vi "Test App Error Handler is Configured for Immediate Parent of Nested Process.vi"(8 "error in (no error)":errorcluster, 11 "Rig Test In":refnum<class "Application Test.lvclass">) -> (0 "error out":errorcluster, 3 "Rig Test Out":refnum<class "Application Test.lvclass">)   [LabVIEW 2020, in "Application Test.lvclass"]
uses:
  Application Test.lvclass
  Framework/Process/Process.lvclass
  Mock Error Handler/Mock Error Handler.lvclass
  Mock Process/Mock Process.lvclass
  Framework/Application/Application.lvclass
  <vilib>/Asteme/LUnit/Test Case.lvclass
  C:/Users/anton/Documents/GitHub/Triarc-Framework/source/Framework/Process/Process.lvclass
  C:/Users/anton/Documents/GitHub/Triarc-Framework/source/Framework/Base/Base.lvclass
  C:/Users/anton/Documents/GitHub/Triarc-Framework/source/Framework/Error Handler Interface/Error Handler Interface.lvclass
  C:/Users/anton/Documents/GitHub/Triarc-Framework/source/Framework/Logging/Logging.lvclass
  C:/Users/anton/Documents/GitHub/Triarc-Framework/source/Framework/Application/Application.lvclass
  C:/Users/anton/Documents/GitHub/Triarc-Framework/source/Framework Test/Process Test/Process Test.lvclass
  C:/Users/anton/Documents/GitHub/Triarc-Framework/source/Framework Test/Base Class Test/Base Test.lvclass
  C:/Program Files (x86)/National Instruments/LabVIEW 2020/vi.lib/Asteme/LUnit/Test Case.lvclass
  C:/Users/anton/Documents/GitHub/Triarc-Framework/source/Framework Test/Application Test/Application Test.lvclass
  C:/Users/anton/Documents/GitHub/Triarc-Framework/source/Framework Test/Mock Process/Mock Process.lvclass
  C:/Users/anton/Documents/GitHub/Triarc-Framework/source/Framework/Helper Loop/Helper Loop.lvclass
  C:/Users/anton/Documents/GitHub/Triarc-Framework/source/Framework Test/Mock Error Handler/Mock Error Handler.lvclass
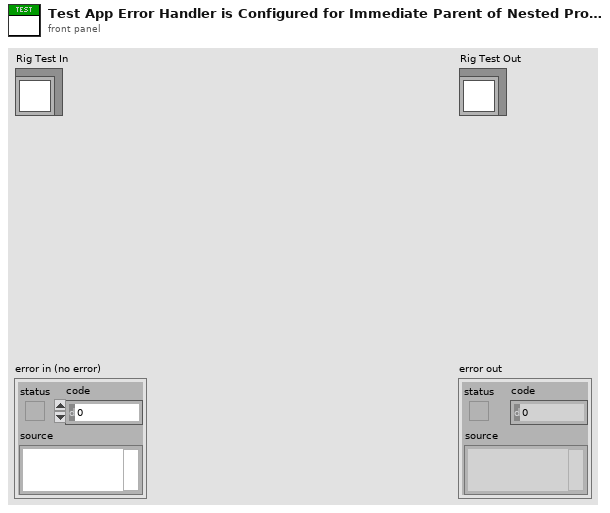
[diagram p1: front panel]
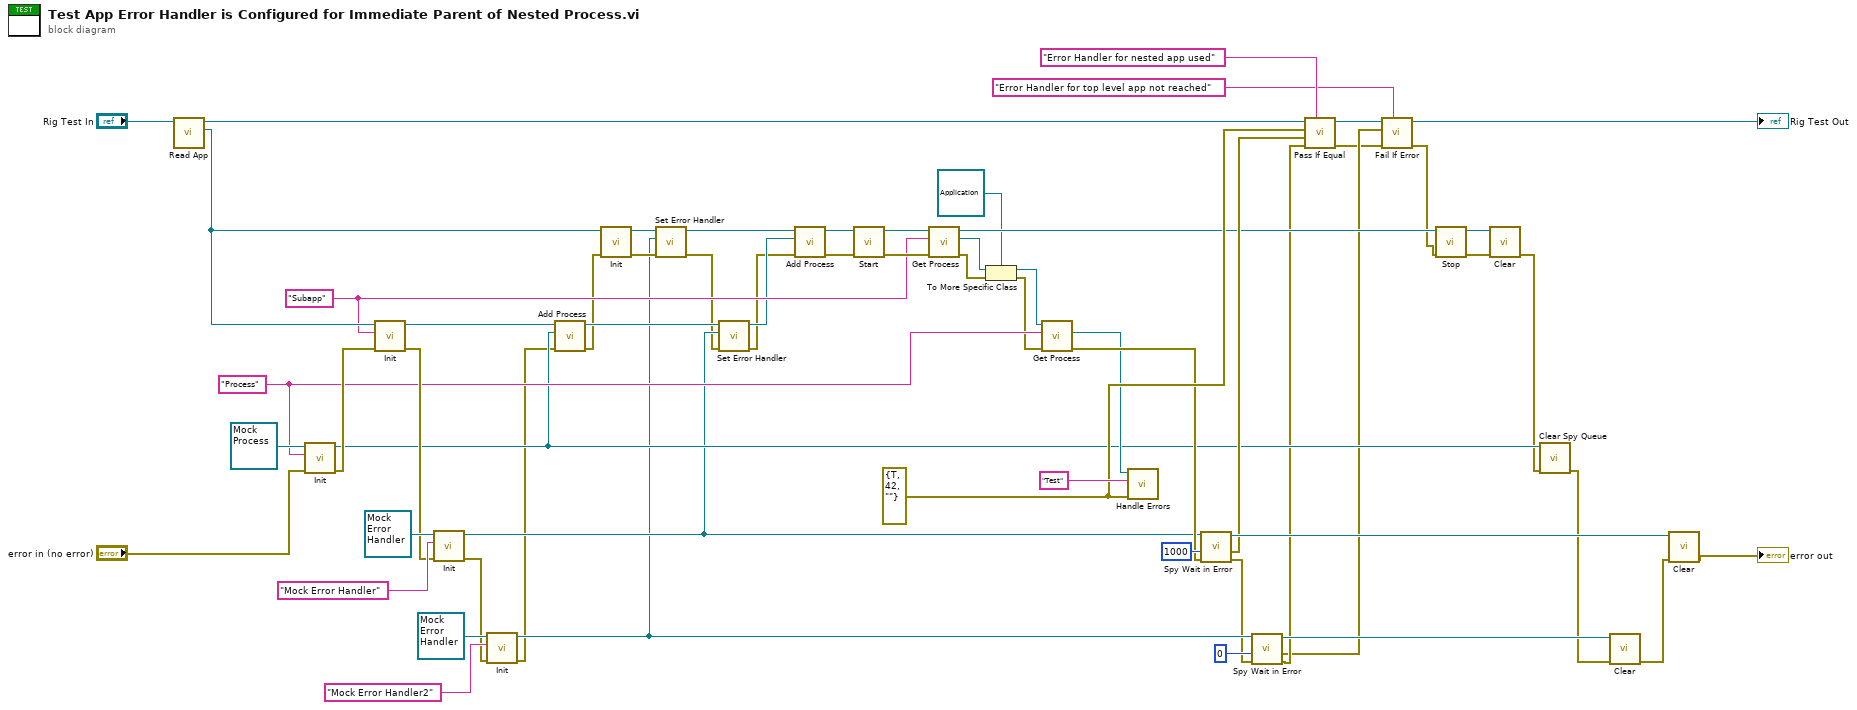
[diagram p0: block diagram]
diagram:
  w31 = "Subapp" ("Name")
  w49 = errorcluster {"status"=TRUE, "code"=42, "source"=""} ("error in (no error)")
  w44 = "Process" ("Name")
  n1 = call "Read App.vi"("Application Test In"="Rig Test In") -> ("App out"=w36:refnum<class "Application.lvclass">, "Application Test Out"=w57:refnum<class "Application Test.lvclass">)  [unwired: 8 in, 1 out]
  n2 = call-dynamic "Init.vi"("error in (no error)"="error in (no error)", "Name"=w44, "Mock Process In"=refnum<class "Mock Process.lvclass"> refnum ("Mock Process.lvclass")) -> ("error out"=w53:errorcluster, "Mock Process Out"=w42:refnum<class "Mock Process.lvclass">)  [unwired: 7 in]
  n3 = call-dynamic "Init.vi"("error in (no error)"=w53, "Name"=w31, "Process In"=w36) -> ("error out"=w52:errorcluster, "Process Out"=w60:refnum<class "Application.lvclass">)  [unwired: 7 in]
  n4 = call-dynamic "Init.vi"("error in (no error)"=w52, "Name"="Mock Error Handler", "Mock Error Handler In"=refnum<class "Mock Error Handler.lvclass"> refnum ("Mock Error Handler.lvclass")) -> ("error out"=w12:errorcluster, "Mock Error Handler Out"=w21:refnum<class "Mock Error Handler.lvclass">)  [unwired: 7 in]
  n5 = call-dynamic "Init.vi"("error in (no error)"=w12, "Name"="Mock Error Handler2", "Mock Error Handler In"=refnum<class "Mock Error Handler.lvclass"> refnum ("Mock Error Handler.lvclass")) -> ("error out"=w11:errorcluster, "Mock Error Handler Out"=w13:refnum<class "Mock Error Handler.lvclass">)  [unwired: 7 in]
  n6 = call "Add Process.vi"("error in (no error)"=w11, "Process"=w42, "Rig In"=w60) -> ("error out"=w20:errorcluster, "Rig Out"=w23:refnum<class "Application.lvclass">)  [unwired: 7 in]
  n7 = call-dynamic "Init.vi"("error in (no error)"=w20, "Process In"=w36) -> ("error out"=w33:errorcluster, "Process Out"=w25:refnum<class "Application.lvclass">)  [unwired: 8 in]
  n8 = call "Set Error Handler.vi"("error in (no error)"=w33, "Error Handler"=w13, "Process In"=w25) -> ("error out"=w19:errorcluster, "Process Out"=w24:refnum<class "Application.lvclass">)  [unwired: 7 in]
  n9 = call "Set Error Handler.vi"("error in (no error)"=w19, "Error Handler"=w21, "Process In"=w23) -> ("error out"=w18:errorcluster, "Process Out"=w22:refnum<class "Application.lvclass">)  [unwired: 7 in]
  n10 = call "Add Process.vi"("error in (no error)"=w18, "Process"=w22, "Rig In"=w24) -> ("error out"=w41:errorcluster, "Rig Out"=w38:refnum<class "Application.lvclass">)  [unwired: 7 in]
  n11 = call "Start.vi"("error in (no error)"=w41, "Process In"=w38) -> ("error out"=w39:errorcluster, "Process Out"=w37:refnum<class "Application.lvclass">)  [unwired: 8 in]
  n12 = call "Get Process.vi"("error in (no error)"=w39, "Process Name"=w31, "Rig In"=w37) -> ("error out"=w28:errorcluster, "App Process"=w29:refnum<class "Process.lvclass">, "Rig Out"=w32:refnum<class "Application.lvclass">)  [unwired: 6 in]
  n13 = To More Specific Class(target class=refnum<class "Application.lvclass"> refnum ("Rig Out"), reference=w29, error in=w28) -> (specific class reference=w26:refnum<class "Application.lvclass">, error out=w27:errorcluster)
  n14 = call "Get Process.vi"("error in (no error)"=w27, "Process Name"=w44, "Rig In"=w26) -> ("error out"=w45:errorcluster, "App Process"=w43:refnum<class "Process.lvclass">)  [unwired: 6 in, 1 out]
  n15 = call-dynamic "Handle Errors.vi"("error in (no error)"=w49, "Location"="Test", "Process In"=w43) -> ()  [unwired: 7 in, 2 out]
  n16 = call "Spy Wait in Error.vi"("error in (no error)"=w45, "timeout in ms (-1)"=1000, "Mock Error Handler In"=w21) -> ("error out"=w7:errorcluster, "Errors"=w47:errorcluster, "Mock Error Handler Out"=w48:refnum<class "Mock Error Handler.lvclass">)  [unwired: 4 in, 2 out]
  n17 = call "Spy Wait in Error.vi"("error in (no error)"=w7, "timeout in ms (-1)"=0, "Mock Error Handler In"=w13) -> ("error out"=w6:errorcluster, "Errors"=w5:errorcluster, "Mock Error Handler Out"=w16:refnum<class "Mock Error Handler.lvclass">)  [unwired: 4 in, 2 out]
  n18 = call <vilib>:"Pass If Equal.vi"("Description"="Error Handler for nested app used", "error in (no error)"=w6, "Actual"=w47, "Expected"=w49, "Test Case In"=w57) -> ("error out"=w4:errorcluster, "Test Case Out"=w9:refnum<class "Application Test.lvclass">)  [unwired: 5 in]
  n19 = call <vilib>:"Fail If Error.vi"("Description"="Error Handler for top level app not reached", "error in (no error)"=w4, "Assert error"=w5, "Test Case In"=w9) -> ("error out"=w10:errorcluster, "Test Case Out"=→"Rig Test Out":refnum<class "Application Test.lvclass">)  [unwired: 6 in]
  n20 = call "Stop.vi"("error in (no error)"=w10, "Process In"=w32) -> ("error out"=w35:errorcluster, "Process Out"=w40:refnum<class "Application.lvclass">)  [unwired: 7 in, 1 out]
  n21 = call-dynamic "Clear.vi"("error in (no error)"=w35, "Application In"=w40) -> ("error out"=w34:errorcluster)  [unwired: 8 in, 1 out]
  n22 = call-dynamic "Clear Spy Queue.vi"("error in (no error)"=w34, "Mock Process In"=w42) -> ("error out"=w2:errorcluster)  [unwired: 8 in, 1 out]
  n23 = call-dynamic "Clear.vi"("error in (no error)"=w2, "Mock Process In"=w16) -> ("error out"=w1:errorcluster)  [unwired: 8 in, 1 out]
  n24 = call-dynamic "Clear.vi"("error in (no error)"=w1, "Mock Process In"=w48) -> ("error out"=→"error out":errorcluster)  [unwired: 8 in, 1 out]
